vi "Plot resize horizontal textwidth.vi"(8 "error in (no error)":errorcluster, 11 "top array":refnum<vi>) -> (0 "error out":errorcluster, 2 "full textbox width":i16)   [LabVIEW 2021, in "RocketPlot.lvlib"]
uses:
  RocketPlot.lvlib
  TypeDefs/Plot top row.ctl
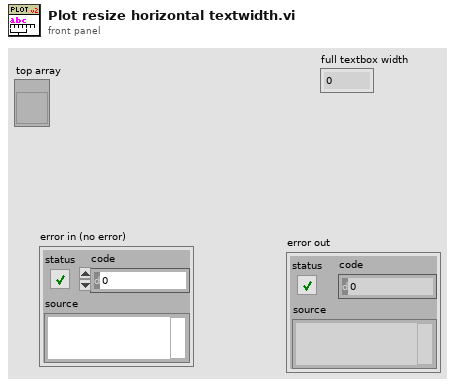
[diagram p1: front panel]
types:
  T1 = typedef "Plot top row.ctl" = cluster{"PID":string, "index":i32, "PID color":u32, "right axis?":bool, "Flatline?":bool, "Numeric color":u32, "Data":string, "Flat":string}
  T2 = cluster{"left":i16, "top":i16, "right":i16, "bottom":i16}
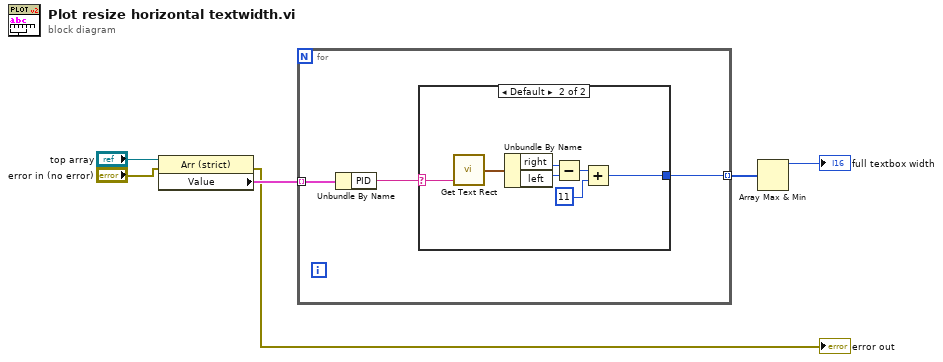
[diagram p0: block diagram]
diagram:
  n1 = property class="Arr (strict)"(reference="top array", error in="error in (no error)") -> (error out=→"error out":errorcluster, "Value"=w4:T1[])  [unwired: 1 out]
  n2 = for {
    tunnel: [w9] -> w6 mode=indexing
    tunnel: w4 -> [w8] mode=indexing
    n3 = Unbundle By Name(w8) -> ("PID"=w7:string)
    n4 = case shown="Default" w7 {
      selector: w7 -> [_ w10]
      tunnel: [_ w11] -> w9
      frame "" {
      }
      frame Default {
        n5 = call <vilib>:"Get Text Rect.vi"("text"=w10) -> ("rect"=w12:T2)  [unwired: 8 in]
        n6 = Unbundle By Name(w12) -> ("right"=w13:i16, "left"=w14:i16)
        n7 = Subtract(x=w13, y=w14) -> (x-y=w15:i16)
        n8 = Add(x=w15, y=i16 11) -> (x+y=w11:i16)
      }
    }
  }
  n9 = Array Max & Min(array=w6) -> (max value=→"full textbox width":i16)  [unwired: 3 out]
